vi "sc5511a_list_buffer_read.vi"(0 "deviceHandle":u32 format="%.0x", 2 "address":u32, 5 "error in":errorcluster) -> (14 "deviceHandle":u32 format="%.0x", 16 "frequency":u64, 19 "error out":errorcluster)   [LabVIEW 2010]
uses:
  sc5511a.dll
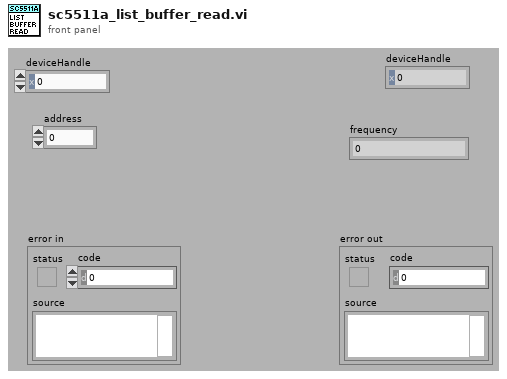
[diagram p1: front panel]
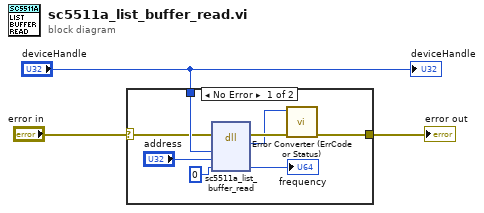
[diagram p0: block diagram]
diagram:
  n1 = case shown="No Error" "error in" {
    selector: "error in" -> [w4 w12]
    tunnel: [w11 w12] -> w3
    tunnel: "deviceHandle" -> [w8 _]
    frame No Error {
      n2 = dll-call lib="sc5511a.dll" fn="sc5511a_list_buffer_read"(error in=w4, "deviceHandle"=w8, "address"="address", "frequency"=u64 0) -> (error out=w10:errorcluster, "return type"=w9:i32, "frequency"=→"frequency":u64)  [unwired: 4 in, 1 out]
      n3 = call "Error Converter (ErrCode or Status).vi"("error in (no error)"=w10, "error code"=w9) -> ("error out"=w11:errorcluster)  [unwired: 9 in]
    }
    frame Error {
    }
  }
  "error out" <- w3
  "deviceHandle" <- "deviceHandle"
